vi "ERIO RT Setup AWS.vi"(8 "error in (no error)":errorcluster, 10 "Supervisory Variables":T1={"Alarm Threshold"=0.0, "Shutdown"=FALSE, "Enable SNS Alarm"=FALSE, "Enable SNS Stage Notification"=FALSE, "Enable SQS Notification"=FALSE, "Enable S3 TDMS Signal Capture"=FALSE, "Enable SystemLink Signal Capture"=FALSE, "Capture Signal"=FALSE, "Server Update"=FALSE, "AWS Access Key"="AKIAINLDO2Y2PDFEWDOQ", "AWS Secret Key"="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", "Phone Number"="+15037066913", "Region"=enum."us-west-2", "AWS SQS Queue"="mynicloud-demotest2", "AWS S3 Bucket"="mynicloud-demotest2"}, 11 "AWS Variables In":T3) -> (0 "error out":errorcluster, 3 "AWS Variables Out":T3)   [LabVIEW 2017]
doc: "Check to see if AWS resources have been setup. If not then set them up. \n\nJames Tillett P.E.\nEndeavor Engineering Inc.\nwww.endeavoreng.com"
uses:
  Controls/ERIO AWS Toolkit Variables.ctl
  <vilib>/AWS Toolkit/SQS/Queue/Queue.lvclass
  <vilib>/AWS Toolkit/SNS/Phone Number/Phone Number.lvclass
  <vilib>/AWS Toolkit/S3/Bucket/Bucket.lvclass
  Controls/ERIO Supervisory Variables.ctl
  <vilib>/AWS Toolkit/Core/HTTP Request/Region.ctl
  <vilib>/AWS Toolkit/Core/HTTP Request/AWS Credentials.ctl
  <vilib>/AWS Toolkit/Core/HTTP Request/HTTP Request.lvclass
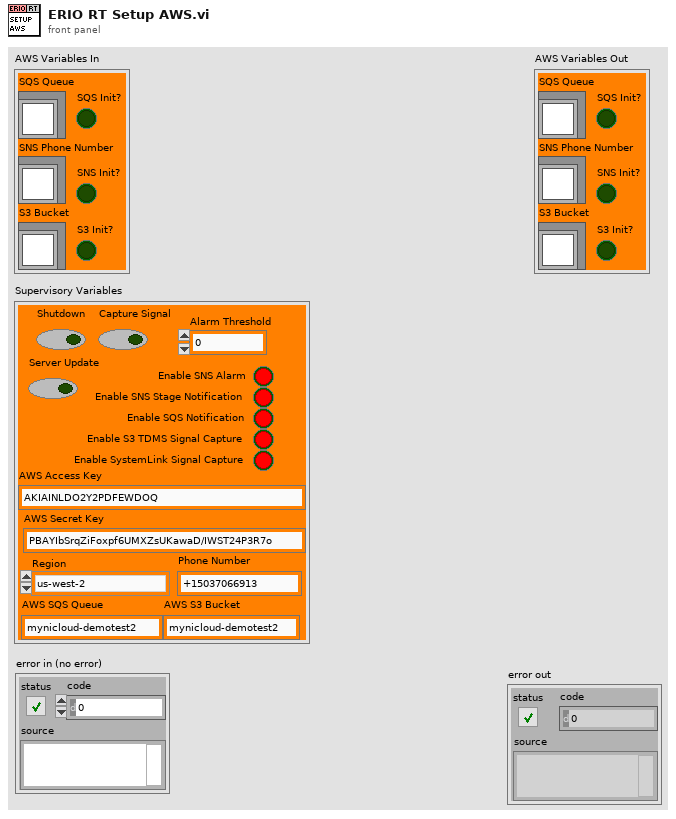
[diagram p1: front panel]
types:
  T1 = typedef "ERIO Supervisory Variables.ctl" = cluster{"Alarm Threshold":dbl, "Shutdown":bool, "Enable SNS Alarm":bool, "Enable SNS Stage Notification":bool, "Enable SQS Notification":bool, "Enable S3 TDMS Signal Capture":bool, "Enable SystemLink Signal Capture":bool, "Capture Signal":bool, "Server Update":bool, "AWS Access Key":string, "AWS Secret Key":string, "Phone Number":string, "Region":T2, "AWS SQS Queue":string, "AWS S3 Bucket":string}
  T2 = typedef "NI_AWS_Core.lvlib/HTTP Request.lvclass/Region.ctl" = enum16{"us-east-1", "us-east-2", "us-west-1", "us-west-2", "ap-northeast-1", "ap-northeast-2", "ap-southeast-1", "ap-southeast-2", "ca-central-1", "eu-central-1", "eu-west-1", "eu-west-2", "sa-east-1"}
  T3 = typedef "ERIO AWS Toolkit Variables.ctl" = cluster{"SQS Queue":refnum<class "Queue.lvclass">, "SNS Phone Number":refnum<class "Phone Number.lvclass">, "S3 Bucket":refnum<class "Bucket.lvclass">, "SQS Init?":bool, "S3 Init?":bool, "SNS Init?":bool}
  T4 = typedef "NI_AWS_Core.lvlib/HTTP Request.lvclass/AWS Credentials.ctl" = cluster{"Access Key":string, "Secret Key":string}
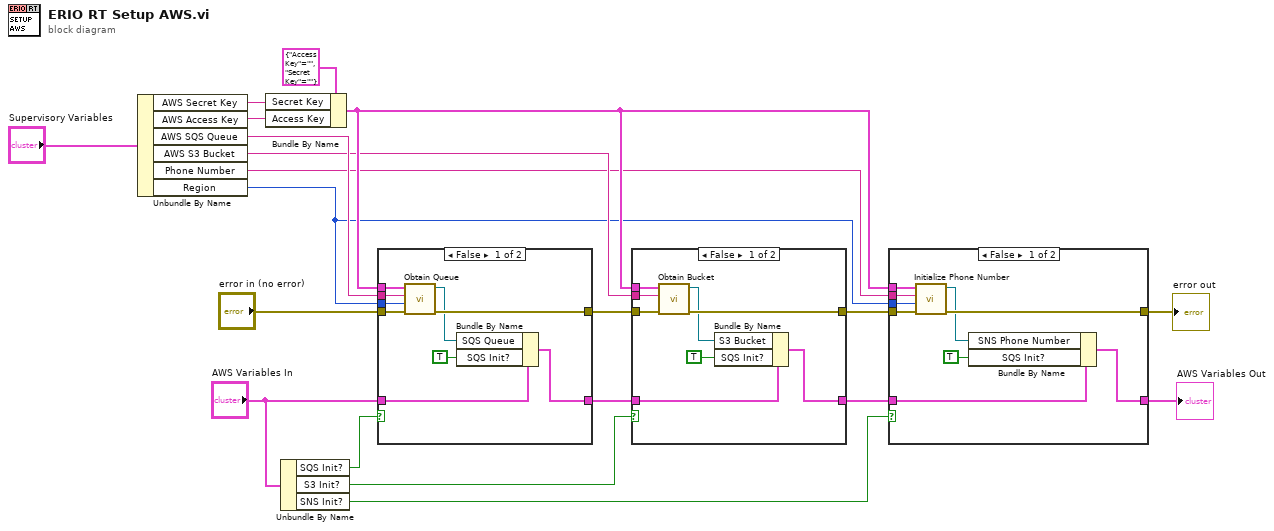
[diagram p0: block diagram]
diagram:
  n1 = Unbundle By Name("Supervisory Variables") -> ("AWS Secret Key"=w15:string, "AWS Access Key"=w14:string, "AWS SQS Queue"=w13:string, "AWS S3 Bucket"=w9:string, "Phone Number"=w7:string, "Region"=w1:T2)
  n2 = Bundle By Name(cluster=T4 {"Access Key"="", "Secret Key"=""} ("AWS Credentials"), "Secret Key"=w15, "Access Key"=w14) -> (w10:T4)
  n3 = Unbundle By Name("AWS Variables In") -> ("SQS Init?"=w20:bool, "S3 Init?"=w3:bool, "SNS Init?"=w2:bool)
  n4 = case shown="False" w20 {
    tunnel: "AWS Variables In" -> [w24 w31]
    tunnel: w10 -> [w29 _]
    tunnel: "error in (no error)" -> [w28 w30]
    tunnel: w13 -> [w27 _]
    tunnel: w1 -> [w26 _]
    tunnel: [w25 w30] -> w8
    tunnel: [w21 w31] -> w12
    frame False {
      n5 = call <vilib>:"Obtain Queue.vi"("error in (no error)"=w28, "Region"=w26, "Name"=w27, "AWS Credentials"=w29) -> ("error out"=w25:errorcluster, "SQS"=w23:refnum<class "Queue.lvclass">)  [unwired: 6 in]
      n6 = Bundle By Name(cluster=w24, "SQS Queue"=w23, "SQS Init?"=TRUE) -> (w21:T3)
    }
    frame True {
    }
  }
  n7 = case shown="False" w3 {
    tunnel: w12 -> [w35 w41]
    tunnel: w10 -> [w39 _]
    tunnel: w8 -> [w38 w40]
    tunnel: w9 -> [w37 _]
    tunnel: [w36 w40] -> w6
    tunnel: [w32 w41] -> w11
    frame False {
      n8 = call <vilib>:"Obtain Bucket.vi"("error in (no error)"=w38, "Bucket name"=w37, "AWS Credentials"=w39) -> ("error out"=w36:errorcluster, "Bucket"=w34:refnum<class "Bucket.lvclass">)  [unwired: 7 in]
      n9 = Bundle By Name(cluster=w35, "S3 Bucket"=w34, "SQS Init?"=TRUE) -> (w32:T3)
    }
    frame True {
    }
  }
  n10 = case shown="False" w2 {
    tunnel: w11 -> [w45 w52]
    tunnel: w10 -> [w50 _]
    tunnel: w6 -> [w49 w51]
    tunnel: w7 -> [w48 _]
    tunnel: w1 -> [w47 _]
    tunnel: [w46 w51] -> w5
    tunnel: [w42 w52] -> w4
    frame False {
      n11 = call <vilib>:"Initialize Phone Number.vi"("error in (no error)"=w49, "Region"=w47, "Phone Number"=w48, "AWS Credentials"=w50) -> ("error out"=w46:errorcluster, "Phone Number"=w44:refnum<class "Phone Number.lvclass">)  [unwired: 6 in]
      n12 = Bundle By Name(cluster=w45, "SNS Phone Number"=w44, "SQS Init?"=TRUE) -> (w42:T3)
    }
    frame True {
    }
  }
  "error out" <- w5
  "AWS Variables Out" <- w4
